vi "M-686 Wait for Motion.vi"(0 "VISA Ref":refnum<visa-resource-name>, 7 "Timeout (s)":i32=5, 11 "Error In":errorcluster) -> (4 "VISA Ref Dup":refnum<visa-resource-name>, 15 "Error Out":errorcluster)   [LabVIEW 2020]
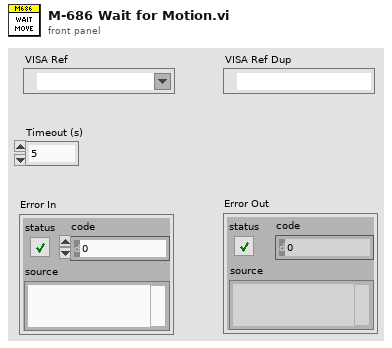
[diagram p1: front panel]
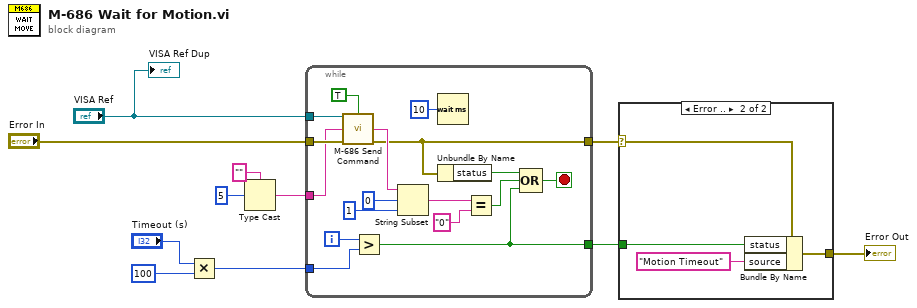
[diagram p0: block diagram]
diagram:
  n1 = Multiply(x="Timeout (s)", y=100) -> (x*y=w5:i32)
  n2 = Type Cast(type="", x=u8 5) -> (*(type *) &x=w9:string)
  n3 = while {
    tunnel: "VISA Ref" -> [w27]
    tunnel: "Error In" -> [w26]
    tunnel: w9 -> [w25]
    tunnel: w5 -> [w15]
    tunnel: [w13] -> w3
    tunnel: [w12] -> w2
    i -> [w16]
    stop <- w14 stop-if-true
    n4 = call "M-686 Send Command.vi"("VISA Ref"=w27, "Wait for Reply (T)"=TRUE, "Command"=w25, "Error In"=w26) -> ("Reply"=w24:string, "Error Out"=w13:errorcluster)  [unwired: 8 in, 2 out]
    n5 = Greater?(x=w16, y=w15) -> (0:w12:bool)
    n6 = String Subset(string=w24, offset (0)=0, length (rest)=1 ("length (rest)")) -> (substring=w21:string)
    n7 = Wait (ms)(milliseconds to wait=u32 10) -> ()  [unwired: 1 out]
    n8 = Unbundle By Name(w13) -> ("status"=w18:bool)
    n9 = Equal?(x=w21, y="0") -> (x = y?=w17:bool)
    n10 = Compound Arithmetic op=OR(w18, w17, w12) -> (w14:bool)
  }
  n11 = case shown="Error .." w3 {
    selector: w3 -> [w29 w33]
    tunnel: w2 -> [_ w32]
    tunnel: [w29 w30] -> w1
    frame No Error {
    }
    frame Error {
      n12 = Bundle By Name(cluster=w33, "status"=w32, "source"="Motion Timeout") -> (w30:errorcluster)
    }
  }
  "Error Out" <- w1
  "VISA Ref Dup" <- "VISA Ref"
